vi "Split Path.vi"(11 "Item Path":string) -> (3 "Item Name":string, 5 "Parent Path":string)   [LabVIEW 2012, in "Negentropic IDE.lvlib"]
uses:
  Negentropic IDE.lvlib
  <vilib>/regexp/Match Regular Expression.xnode
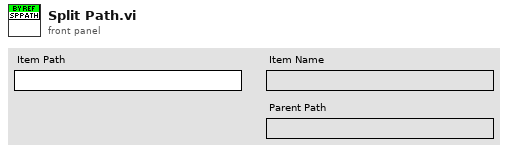
[diagram p1: front panel]
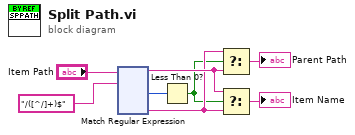
[diagram p0: block diagram]
diagram:
  n1 = xnode "Match Regular Expression"("input string"="Item Path", "regular expression"="/([^/]+)$") -> ("before match"=w4:string, "offset past match"=w6:i32, "submatch 1"=w3:string)  [unwired: 4 in, 3 out]
  n2 = Less Than 0?(x=w6) -> (x < 0?=w2:bool)
  n3 = Select(t=w3, s=w2, f=w4) -> (s? t:f=→"Parent Path":string)
  n4 = Select(t=w4, s=w2, f=w3) -> (s? t:f=→"Item Name":string)
